vi "VIE.Module.Queued Message Handler.dqClass_setModifiedData.vi"(0 "reference":T2, 1 "data (unmodified)":T1, 2 "data":T1, 5 "error in (no error)":errorcluster) -> (14 "duplicate reference":T2, 19 "error out":errorcluster)   [LabVIEW 2010, in "VIE.Module.Queued Message Handler.QueuedMessageHandler.dqGOOPClass.lvlib"]
doc: "This VI writes the data of the dqGOOP object and unlocks it for write access"
uses:
  VIE.Module.Queued Message Handler.QueuedMessageHandler.dqGOOPClass.lvlib
  VIE.Module.Queued Message Handler.dqClass_ObjectReference.ctl
  VIE.Module.Queued Message Handler.dqClass_ObjectData.ctl
panel:
  in  "queue (default)":refnum<queue>
  # "Copyright (C) 2004 DataAct Incorporated"
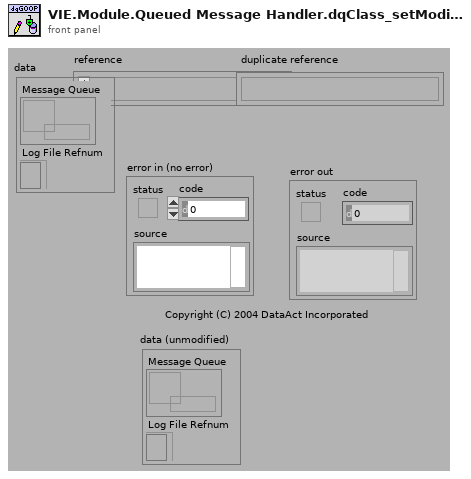
[diagram p1: front panel]
types:
  T1 = typedef "VIE.Module.Queued Message Handler.QueuedMessageHandler.dqGOOPClass.lvlib/VIE.Module.Queued Message Handler.dqClass_ObjectData.ctl" = cluster{"Message Queue":refnum<queue>, "Log File Refnum":refnum<file>}
  T2 = typedef "VIE.Module.Queued Message Handler.QueuedMessageHandler.dqGOOPClass.lvlib/VIE.Module.Queued Message Handler.dqClass_ObjectReference.ctl" = refnum<k1>
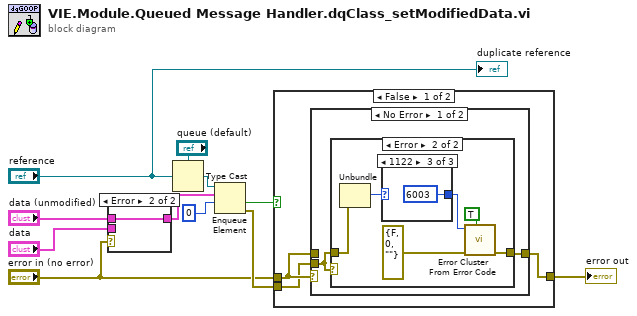
[diagram p0: block diagram]
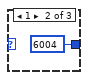
[diagram p5: hidden frame]
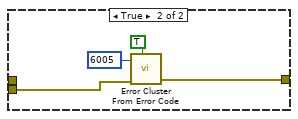
[diagram p7: hidden frame]
diagram:
  n1 = case shown="Error" "error in (no error)" {
    tunnel: [w12 w13] -> w5
    tunnel: "data (unmodified)" -> [_ w13]
    tunnel: "data" -> [w12 _]
    frame No Error {
    }
    frame Error {
    }
  }
  n2 = Type Cast(type="queue (default)", x="reference") -> (*(type *) &x=w2:refnum<queue>)
  n3 = Enqueue Element(queue=w2, element=w5, timeout in ms (-1)=0 ("timeout in ms (0)")) -> (timed out?=w9:bool, error out=w11:errorcluster)  [unwired: 1 in, 1 out]
  n4 = case shown="False" w9 {
    tunnel: "error in (no error)" -> [w16 _]
    tunnel: w11 -> [w15 w31]
    tunnel: [w14 w32] -> w10
    frame False {
      n5 = case shown="No Error" w16 {
        tunnel: [w17 w29] -> w14
        tunnel: w16 -> [_ w29]
        tunnel: w15 -> [w18 _]
        frame No Error {
          n6 = case shown="Error" w18 {
            tunnel: [w19 w20] -> w17
            tunnel: w18 -> [w19 w25]
            frame No Error {
            }
            frame Error {
              n7 = Unbundle(w25) -> ("code"=w24:i32)  [unwired: 2 out]
              n8 = case shown="1122" w24 {
                selector: w24 -> [w26 _ _]
                tunnel: [w26 6004 ("code") 6003 ("code")] -> w22
                frame Default {
                }
                frame 1 {
                }
                frame 1122 {
                }
              }
              n9 = call <vilib>:"Error Cluster From Error Code.vi"("show call chain? (False)"=TRUE, "error in (no error)"=errorcluster {"status"=FALSE, "code"=0, "source"=""} ("error out"), "error code (0)"=w22) -> ("error out"=w20:errorcluster)  [unwired: 6 in]
            }
          }
        }
        frame Error {
        }
      }
    }
    frame True {
      n10 = call <vilib>:"Error Cluster From Error Code.vi"("show call chain? (False)"=TRUE, "error in (no error)"=w31, "error code (0)"=6005 ("code")) -> ("error out"=w32:errorcluster)  [unwired: 6 in]
    }
  }
  "error out" <- w10
  "duplicate reference" <- "reference"
